vi "ParsedivID.vi"(0 "Text in":string, 1 "HTML in":string) -> (2 "Test out":string, 4 "HTML out":string)   [LabVIEW 2018]
doc: "Parses HTML and color codes"
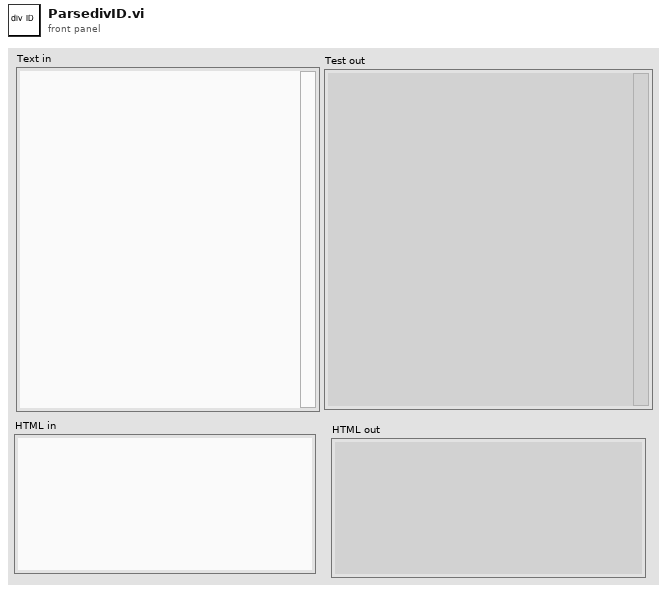
[diagram p1: front panel]
types:
  T1 = cluster{"text color(black)":u32, "result string":string}
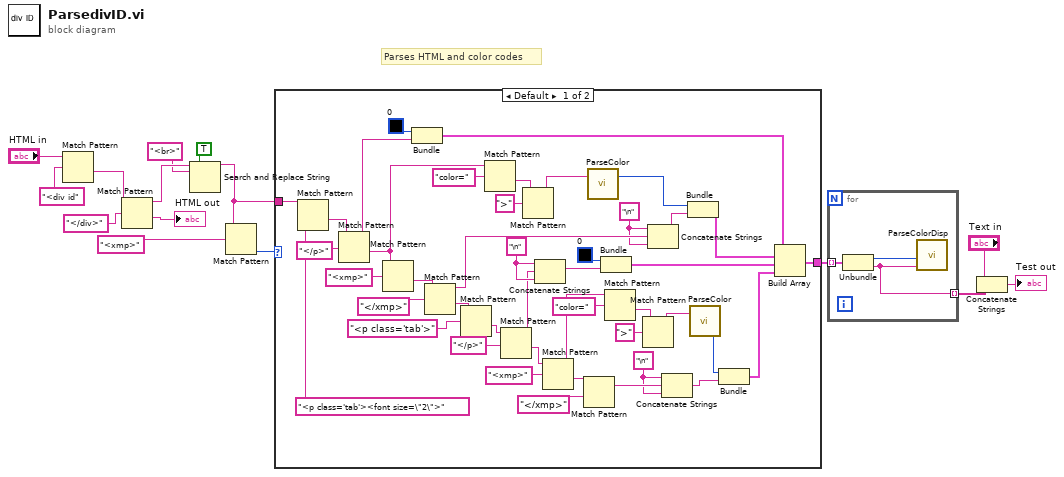
[diagram p0: block diagram]
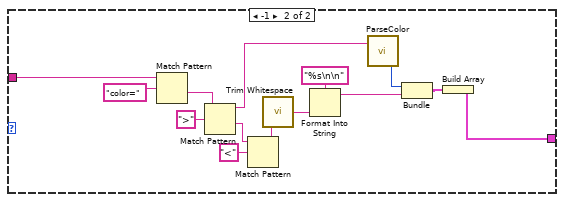
[diagram p2: hidden frame]
diagram:
  # "Parses HTML and color codes"
  n1 = Match Pattern(string="HTML in", regular expression="<div id") -> (after substring=w8:string)  [unwired: 1 in, 3 out]
  n2 = Match Pattern(string=w8, regular expression="</div>") -> (before substring=w14:string, after substring=→"HTML out":string)  [unwired: 1 in, 2 out]
  n3 = Search and Replace String(replace all?=TRUE ("replace all? (F)"), input string=w14, search string="<br>") -> (result string=w15:string)  [unwired: 5 in, 3 out]
  n4 = Match Pattern(string=w15, regular expression="<xmp>") -> (offset past match=w11:i32)  [unwired: 1 in, 3 out]
  n5 = case shown="Default" w11 {
    tunnel: w15 -> [w59 w71]
    tunnel: [w19 w60] -> w3
    frame Default {
      w18 = "\n" ("regular expression")
      w31 = "\n" ("regular expression")
      w44 = "\n" ("regular expression")
      n6 = Match Pattern(string=w59, regular expression="<p class='tab'><font size=\"2\">") -> (after substring=w58:string)  [unwired: 1 in, 3 out]
      n7 = Match Pattern(string=w58, regular expression="</p>") -> (before substring=w30:string, after substring=w41:string)  [unwired: 1 in, 2 out]
      n8 = Match Pattern(string=w41, regular expression="<xmp>") -> (after substring=w54:string)  [unwired: 1 in, 3 out]
      n9 = Bundle("text color(black)"=u32 0, "result string"=w30) -> (w28:T1)  [unwired: 1 in]
      n10 = Match Pattern(string=w54, regular expression="</xmp>") -> (before substring=w53:string, after substring=w52:string)  [unwired: 1 in, 2 out]
      n11 = Match Pattern(string=w52, regular expression="<p class='tab'>") -> (after substring=w50:string)  [unwired: 1 in, 3 out]
      n12 = Match Pattern(string=w41, regular expression="color=") -> (after substring=w39:string)  [unwired: 1 in, 3 out]
      n13 = Match Pattern(string=w50, regular expression="</p>") -> (before substring=w17:string, after substring=w45:string)  [unwired: 1 in, 2 out]
      n14 = Match Pattern(string=w39, regular expression=">") -> (before substring=w38:string)  [unwired: 1 in, 3 out]
      n15 = Concatenate Strings(w18, w17, w18) -> (w16:string)
      n16 = Match Pattern(string=w45, regular expression="<xmp>") -> (before substring=w33:string, after substring=w48:string)  [unwired: 1 in, 2 out]
      n17 = Match Pattern(string=w48, regular expression="</xmp>") -> (before substring=w32:string)  [unwired: 1 in, 3 out]
      n18 = call <userlib>:"ParseColor.vi"("HTML in"=w38) -> ("Color"=w26:u32)  [unwired: 2 in]
      n19 = Bundle("text color(black)"=u32 0, w16) -> (w23:cluster{"text color(black)":u32, string})  [unwired: 1 in]
      n20 = Match Pattern(string=w33, regular expression="color=") -> (after substring=w36:string)  [unwired: 1 in, 3 out]
      n21 = Match Pattern(string=w36, regular expression=">") -> (before substring=w37:string)  [unwired: 1 in, 3 out]
      n22 = Concatenate Strings(w44, w53, w44) -> (w27:string)
      n23 = Concatenate Strings(w31, w32, w31) -> (w22:string)
      n24 = Bundle("Color"=w26, w27) -> (w25:cluster{"Color":u32, string})  [unwired: 1 in]
      n25 = call <userlib>:"ParseColor.vi"("HTML in"=w37) -> ("Color"=w21:u32)  [unwired: 2 in]
      n26 = Bundle("Color"=w21, w22) -> (w20:cluster{"Color":u32, string})  [unwired: 1 in]
      n27 = Build Array(w28, w25, w23, w20) -> (w19:cluster{"Color":u32, "result string":string}[])
    }
    frame -1 {
      n28 = Match Pattern(string=w71, regular expression="color=") -> (after substring=w72:string)  [unwired: 1 in, 3 out]
      n29 = Match Pattern(string=w72, regular expression=">") -> (before substring=w66:string, after substring=w68:string)  [unwired: 1 in, 2 out]
      n30 = Match Pattern(string=w68, regular expression="<") -> (before substring=w67:string)  [unwired: 1 in, 3 out]
      n31 = call <vilib>:"Trim Whitespace.vi"("string"=w67) -> ("trimmed string"=w64:string)  [unwired: 1 in]
      n32 = Format Into String(format string="%s\n\n" ("regular expression"), w64) -> (resulting string=w63:string)  [unwired: 2 in, 1 out]
      n33 = call <userlib>:"ParseColor.vi"("HTML in"=w66) -> ("Color"=w62:u32)  [unwired: 2 in]
      n34 = Bundle("Color"=w62, w63) -> (w61:cluster{"Color":u32, string})  [unwired: 1 in]
      n35 = Build Array(w61) -> (w60:cluster{"Color":u32, string}[])
    }
  }
  n36 = for {
    tunnel: w3 -> [w76] mode=indexing
    tunnel: [w74] -> w2 mode=indexing
    n37 = Unbundle(w76) -> ("Color"=w75:u32, "result string"=w74:string)
    n38 = call <userlib>:"ParseColorDisp.vi"("text"=w74, "text color(black)"=w75) -> ()  [unwired: 2 in, 1 out]
  }
  n39 = Concatenate Strings("Text in", w2) -> (→"Test out":string)
